vi "arrayLength.vi"() -> ()   [LabVIEW 2025]
doc: "Returns the number of elements in the input array."
panel:
  out "array length":dbl
  in  "Array":string[](array[string])
  # "Description: Length of array"
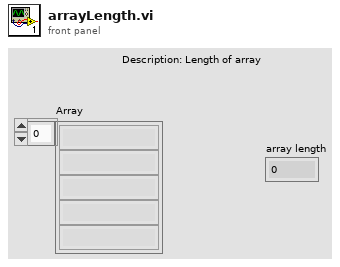
[diagram p1: front panel]
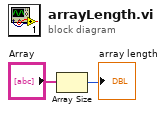
[diagram p0: block diagram]
diagram:
  n1 = Array Size(array="Array") -> (size(s)=→"array length":i32)
